vi "Reset Abort.vi"(8 "error in (no error)":errorcluster, 11 "AbortAPI in":refnum<class "AbortAPI.lvclass">) -> (0 "error out":errorcluster, 3 "AbortAPI out":refnum<class "AbortAPI.lvclass">)   [LabVIEW 2020, in "Volatus.lvlib" / "AbortAPI.lvclass"]
uses:
  AbortAPI.lvclass
  AbortAPI.lvclass/AbortAPI.ctl
  <vilib>/ActorFramework/Message Enqueuer/Message Enqueuer.lvclass/Message Enqueuer.ctl
  <vilib>/ActorFramework/Message Enqueuer/Enqueue.vi
  AbortHandler Messages/Reset Abort Msg/Reset Abort Msg.lvclass
  C:/Program Files (x86)/National Instruments/LabVIEW 2020/vi.lib/ActorFramework/Message/Message.lvclass
  <vilib>/ActorFramework/Message Priority Queue/Priority Enqueue.vi
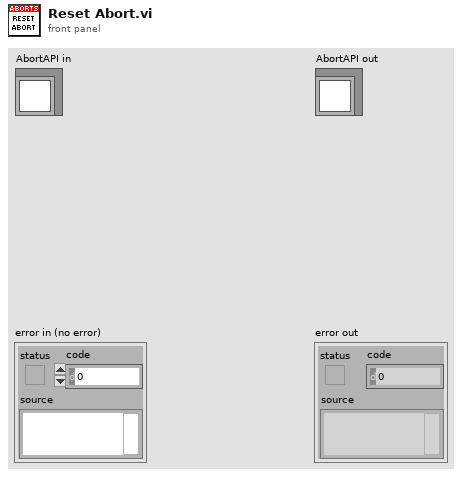
[diagram p1: front panel]
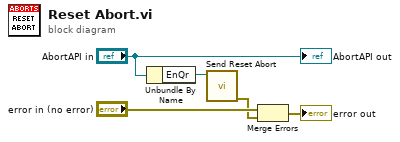
[diagram p0: block diagram]
diagram:
  n1 = Unbundle By Name("AbortAPI in") -> ("EnQr"=w3:refnum<class "Message Enqueuer.lvclass">)
  n2 = call "Send Reset Abort.vi"("Message Enqueuer"=w3) -> ("error out"=w1:errorcluster)  [unwired: 9 in, 1 out]
  n3 = Merge Errors("error in (no error)", w1) -> (→"error out":errorcluster)
  "AbortAPI out" <- "AbortAPI in"
